vi "Test Comparison.vi"(8 "error in (no error)":errorcluster) -> (0 "error out":errorcluster)   [LabVIEW 2020]
uses:
  f8bd0ec0-d98b-4759-ac05-645649cc33d2.vi
  58117923-498f-40ae-a998-025512cbd29e.vi
  <vilib>/numeric/Random Number (Range) DBL.vi
  8602ef81-5ee6-4e9a-b14c-7481c414c614.vi
  59f69eae-4cc6-422f-bea3-69ec6870d71c.vi
  f8bd0ec0-d98b-4759-ac05-645649cc33d2.vi/aaf47be5-b524-48b6-80e6-c7027e155678.vi
  58117923-498f-40ae-a998-025512cbd29e.vi/eacad6df-34c9-4c9e-8205-0119b8e818d4.vi
  <vilib>/addons/_JKI Toolkits/Caraya/classes/Assert/Assert Equal Value and Type_Variant.vi
  <vilib>/addons/_JKI Toolkits/Caraya/classes/Assert/Assert True.vi
  <vilib>/addons/_JKI Toolkits/Caraya/classes/Test/Test.lvclass
  <vilib>/addons/_JKI Toolkits/Caraya/classes/Assert/Assert.lvclass
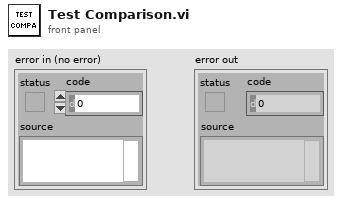
[diagram p1: front panel]
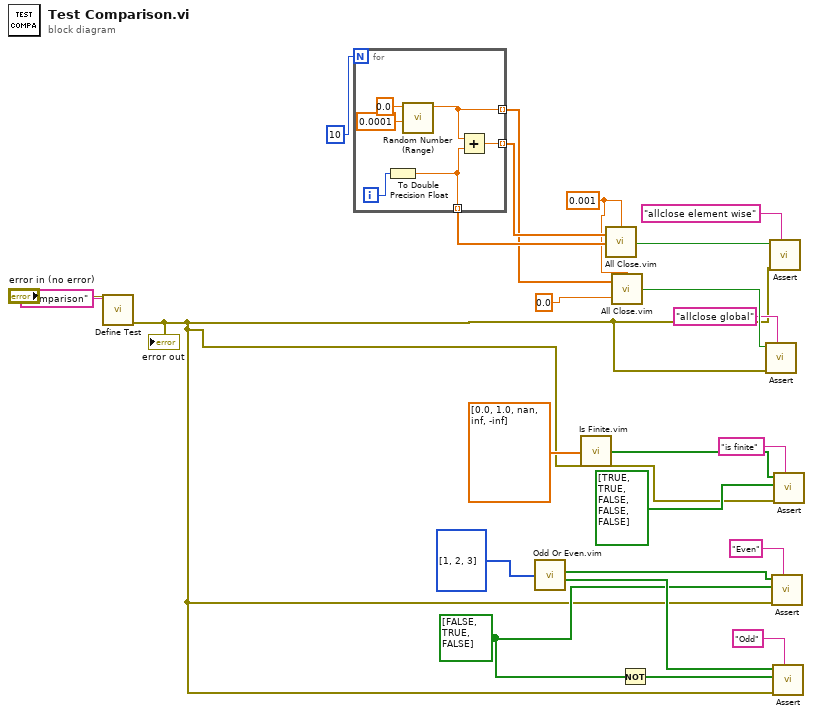
[diagram p0: block diagram]
diagram:
  w4 = bool[] [FALSE, TRUE, FALSE]
  w17 = 0.001 ("Tolerance (1e-12)")
  n1 = call <vilib>:"Define Test.vi"("error in (no error)"="error in (no error)", "Label (VI Title)"="Comparison") -> ("error out"=w2:errorcluster)  [unwired: 9 in]
  "error out" <- w2
  n2 = for {
    N: 10 -> [_]
    tunnel: [w27] -> w22 mode=indexing
    tunnel: [w26] -> w21 mode=indexing
    tunnel: [w25] -> w18 mode=indexing
    i -> [w30]
    n3 = To Double Precision Float(number=w30) -> (double precision float=w26:dbl)
    n4 = call-poly <vilib>:"Random Number (Range).vi"("lower bound (0)"=0.0001, "upper bound (100)"=0.0) -> ("number"=w25:dbl)  [unwired: 9 in]
    n5 = Add(x=w25, y=w26) -> (x+y=w27:dbl)
  }
  n6 = call "Odd Or Even.vim"("Integer"=i64[] [1, 2, 3]) -> ("Odd"=w5:bool[], "Even"=w7:bool[])  [unwired: 6 in]
  n7 = call "Is Finite.vim"("number(s) in"=dbl[] [0.0, 1.0, nan, inf, -inf] ("lower bound (0)")) -> ("Number finite"=w11:bool[])
  n8 = call "All Close.vim"("Tolerance (1e-12)"=w17, "Value A"=w21, "Value B"=w22) -> ("All Close"=w19:bool)
  n9 = call "All Close.vim"("Tolerance (1e-12)"=w17, "Value A"=0.0 ("lower bound (0)"), "Value B"=w18) -> ("All Close"=w16:bool)
  n10 = Not(x=w4) -> (.not. x?=w3:bool[])
  n11 = call-poly <vilib>:"Assert.vi"("Label"="allclose global", "error in (no error)"=w2, "True?"=w16) -> ()  [unwired: 8 in, 1 out]
  n12 = call-poly <vilib>:"Assert.vi"("Label"="allclose element wise", "error in (no error)"=w2, "True?"=w19) -> ()  [unwired: 8 in, 1 out]
  n13 = call-poly <vilib>:"Assert.vi"("Label"="Even", "error in (no error)"=w2, "Y"=w4, "X"=w7) -> ()  [unwired: 7 in, 1 out]
  n14 = call-poly <vilib>:"Assert.vi"("Label"="Odd", "error in (no error)"=w2, "Y"=w3, "X"=w5) -> ()  [unwired: 7 in, 1 out]
  n15 = call-poly <vilib>:"Assert.vi"("Label"="is finite", "error in (no error)"=w2, "Y"=bool[] [TRUE, TRUE, FALSE, FALSE, FALSE], "X"=w11) -> ()  [unwired: 7 in, 1 out]
